vi "G-CLI Example.vi"() -> ()   [LabVIEW 2020]
uses:
  Source/LV Log.lvlib
  <vilib>/Wiresmith Technology/G CLI/CLI Class/CLI.lvclass
  Source/Type Defs/Debug Level.ctl
panel:
  in  "error in (no error)":errorcluster
  in  "Debug Level":T1=enum."DEBUG"
  out "error out":errorcluster
  # "RUN THIS VI FROM COMMAND LINE\nwith:\n\ng-cli \"G-CLI Example.vi\"\n\nYou must ensure that the VI is marked as Run when Opened in Execution Settings"
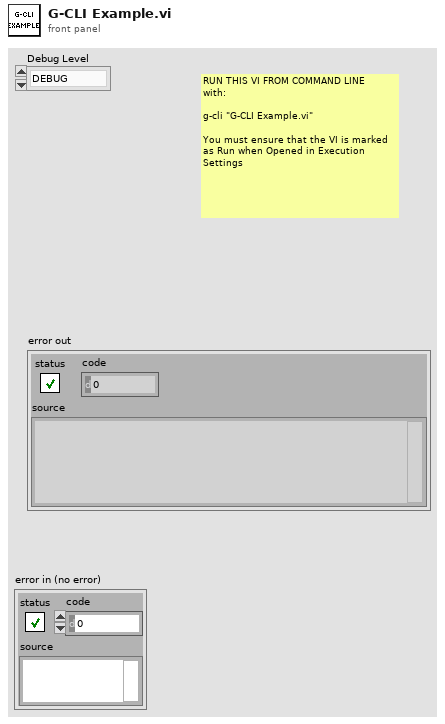
[diagram p1: front panel]
types:
  T1 = typedef "LV Log.lvlib/Debug Level.ctl" = enum16{"DEFAULT", "DEBUG", "INFO", "WARN", "ERROR", "FATAL"}
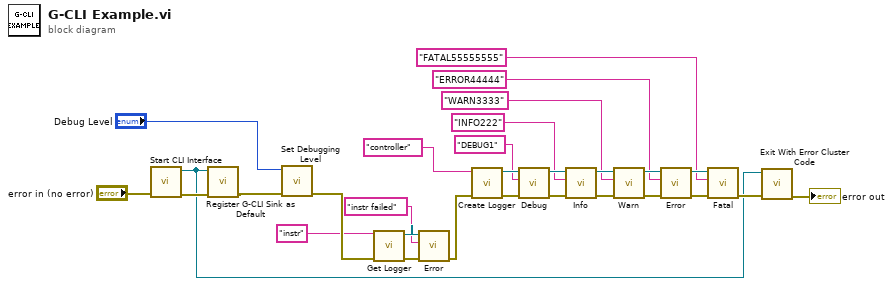
[diagram p0: block diagram]
diagram:
  n1 = call <vilib>:"Start CLI Interface.vi"("error in (no error)"="error in (no error)") -> ("error out"=w4:errorcluster, "CLI out"=w1:refnum<class "CLI.lvclass">)  [unwired: 7 in, 2 out]
  n2 = call "Register G-CLI Sink as Default.vi"("error in (no error)"=w4, "CLI Connection"=w1) -> ("error out"=w6:errorcluster)  [unwired: 9 in]
  n3 = call "Set Debugging Level.vi"("error in (no error)"=w6, "Debug Level in"="Debug Level") -> ("error out"=w27:errorcluster)  [unwired: 9 in]
  n4 = call "Get Logger.vi"("error in (no error)"=w27, "Name"="instr") -> ("error out"=w10:errorcluster, "Logger out"=w9:refnum<class "Logger.lvclass">)  [unwired: 8 in]
  n5 = call "Error.vi"("error in (no error)"=w10, "Log Text"="instr failed", "Logger in"=w9) -> ("error out"=w8:errorcluster)  [unwired: 7 in, 1 out]
  n6 = call "Create Logger.vi"("error in (no error)"=w8, "Name"="controller") -> ("error out"=w25:errorcluster, "Logger out"=w24:refnum<class "Logger.lvclass">)  [unwired: 8 in]
  n7 = call "Debug.vi"("error in (no error)"=w25, "Log Text"="DEBUG1", "Logger in"=w24) -> ("error out"=w22:errorcluster, "Logger out"=w23:refnum<class "Logger.lvclass">)  [unwired: 7 in]
  n8 = call "Info.vi"("error in (no error)"=w22, "Log Text"="INFO222", "Logger in"=w23) -> ("error out"=w21:errorcluster, "Logger out"=w20:refnum<class "Logger.lvclass">)  [unwired: 7 in]
  n9 = call "Warn.vi"("error in (no error)"=w21, "Log Text"="WARN3333", "Logger in"=w20) -> ("error out"=w18:errorcluster, "Logger out"=w19:refnum<class "Logger.lvclass">)  [unwired: 7 in]
  n10 = call "Error.vi"("error in (no error)"=w18, "Log Text"="ERROR44444", "Logger in"=w19) -> ("error out"=w17:errorcluster, "Logger out"=w16:refnum<class "Logger.lvclass">)  [unwired: 7 in]
  n11 = call "Fatal.vi"("error in (no error)"=w17, "Log Text"="FATAL55555555", "Logger in"=w16) -> ("error out"=w3:errorcluster)  [unwired: 7 in, 1 out]
  n12 = call <vilib>:"Exit With Error Cluster Code.vi"("error in (no error)"=w3, "CLI in"=w1) -> ("error out"=→"error out":errorcluster)  [unwired: 9 in]
